vi "Cascade Windows.vi"(7 "Order":T1 items=["List order"=2, "Z order"=4], 8 "error in (no error)":errorcluster, 9 "ChildHwnd[]":u32[](array[numeric]), 10 "Child Count":i32, 11 "Parent Hwnd":i32) -> (0 "error out":errorcluster)   [LabVIEW 2016, in "LV MDI.lvclass"]
doc: "Cascade child windows within the parent window."
uses:
  LV MDI.lvclass
  Typedef/Cascade Order.ctl
  user32.dll
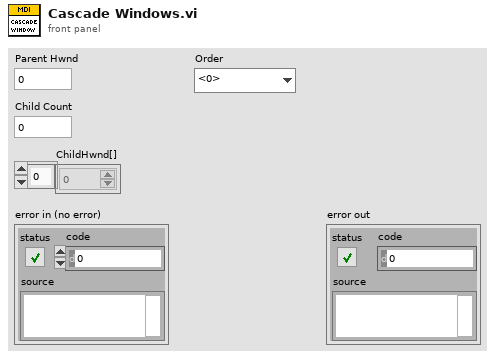
[diagram p1: front panel]
types:
  T1 = typedef "LV MDI.lvclass/Cascade Order.ctl" = u16
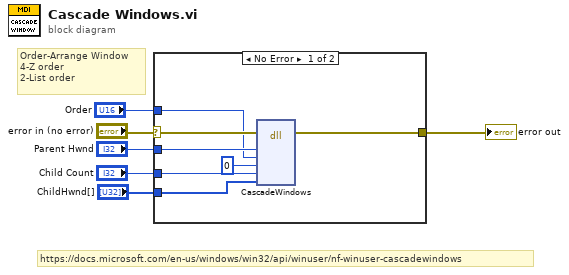
[diagram p0: block diagram]
diagram:
  # "https://docs.microsoft.com/en-us/windows/win32/api/winuser/nf-winuser-cascadewindows"
  # "Order-Arrange Window\n4-Z order\n2-List order"
  n1 = case shown="No Error" "error in (no error)" {
    selector: "error in (no error)" -> [w12 w14]
    tunnel: [w13 w14] -> w6
    tunnel: "Child Count" -> [w11 _]
    tunnel: "Parent Hwnd" -> [w10 _]
    tunnel: "Order" -> [w9 _]
    tunnel: "ChildHwnd[]" -> [w8 _]
    frame No Error {
      n2 = dll-call lib="user32.dll" fn="CascadeWindows"(error in=w12, "hwndParent"=w10, "wHow"=w9, "lpRect"=0 ("wHow"), "cKids"=w11, "lpKids"=w8) -> (error out=w13:errorcluster)  [unwired: 8 in, 1 out]
    }
    frame Error {
    }
  }
  "error out" <- w6
